vi "Elevator Control.vi"(11 "Shooter Elevation PID Gains":T1={"proportional gain (Kc)"=2.5, "integral time (Ti, min)"=0.0, "derivative time (Td, min)"=0.0003} {"derivative time (Td, min)" format="%.5f"; "integral time (Ti, min)" format="%.3f"; "proportional gain (Kc)" format="%.3f"}) -> (2 "Shooter Pot Setpoint":dbl=3.84, 3 "Elevator Output":dbl=-0.06325507999999869)   [LabVIEW 2012]
uses:
  Globals/Shooter Elevation Positons.vi
  Globals/Useful Values.vi
  <vilib>/Rock Robotics/WPI/Joystick/WPI_JoystickGetSetRefNum.vi
  Robot Global Data.vi
  Globals/Log Data.vi
  <vilib>/addons/control/pid/pid.llb/PID (DBL).vi
  <vilib>/addons/control/pid/NI_PID_pid.lvlib
panel:
  out "Shooter Pot Voltage":dbl
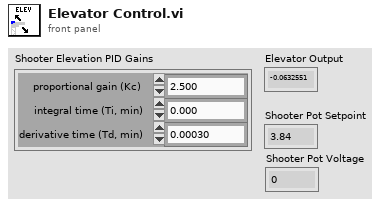
[diagram p1: front panel]
types:
  T1 = cluster{"proportional gain (Kc)":dbl, "integral time (Ti, min)":dbl, "derivative time (Td, min)":dbl}
  T2 = typedef "WPI_AnalogChannelDevRef.ctl" = cluster{"DevStatus":errorcluster, "Analog Module":T3, "Analog Channel":T4}
  T3 = typedef "FPGA_TypedefAnalogModule.ctl" = enum16{"Analog Module 1", "Analog Module 2"}
  T4 = typedef "FPGA_AIChannel.ctl" = enum8{"AI 1", "AI 2", "AI 3", "AI 4", "AI 5", "AI 6", "AI 7", "AI 8", "Invalid"}
  T5 = typedef "WPI_MotorControlDeviceRef.ctl" = cluster{"DeviceStatus":errorcluster, "Type":enum16{"PWM", "CAN"}, "PWM":cluster{"Digital Module":T6, "PWM Channel":T7, "DeadBand":T8}, "CAN":cluster{"Device Number":u8, "Control Mode":T9, "Semaphore":T10, "Max Vout":dbl}, "Invert":bool, "TransformRef":T11, "InvTransformRef":T11}
  T6 = typedef "FPGA_TypedefDigitalModule.ctl" = enum16{"Digital Module 1", "Digital Module 2"}
  T7 = typedef "FPGA_DIOPWMChannel.ctl" = enum8{"PWM 1", "PWM 2", "PWM 3", "PWM 4", "PWM 5", "PWM 6", "PWM 7", "PWM 8", "PWM 9", "PWM 10", "Invalid"}
  T8 = typedef "WPI_PWMDeadband.ctl" = cluster{"Name":string, "maxPositivePwm":i32, "minPositivePwm":i32, "centerPwm":i32, "maxNegativePwm":i32, "minNegativePwm":i32, "angularRange":u16}
  T9 = typedef "WPI_CANJaguar_ControlMode.ctl" = enum8{"Percent VBus", "Current", "Speed", "Position", "Voltage"}
  T10 = typedef "Semaphore RefNum" = refnum<k1>
  T11 = typedef "WPI_PWMTransform_ConPane.ctl" = refnum<vi>
  T12 = typedef "WPI_JoystickDevRef.ctl" = cluster{"Device":T13}
  T13 = typedef "WPI_JoystickDeviceEnum.ctl" = enum16{"USB 1", "USB 2", "USB 3", "USB 4", "Kinect 1", "Kinect 2"}
  T14 = typedef "WPI_JoystickButtonState.ctl" = cluster{"Button 1":bool, "Button 2":bool, "Button 3":bool, "Button 4":bool, "Button 5":bool, "Button 6":bool, "Button 7":bool, "Button 8":bool, "Button 9":bool, "Button 10":bool, "Button 11":bool, "Button 12":bool}
  T15 = typedef "WPI_DriverStationRobotMode2.ctl" = enum16{"Autonomous Disabled", "Autonomous Enabled", "Teleop Disabled", "Teleop Enabled", "Timeout", "Finish", "Test Disabled", "Test Enabled"}
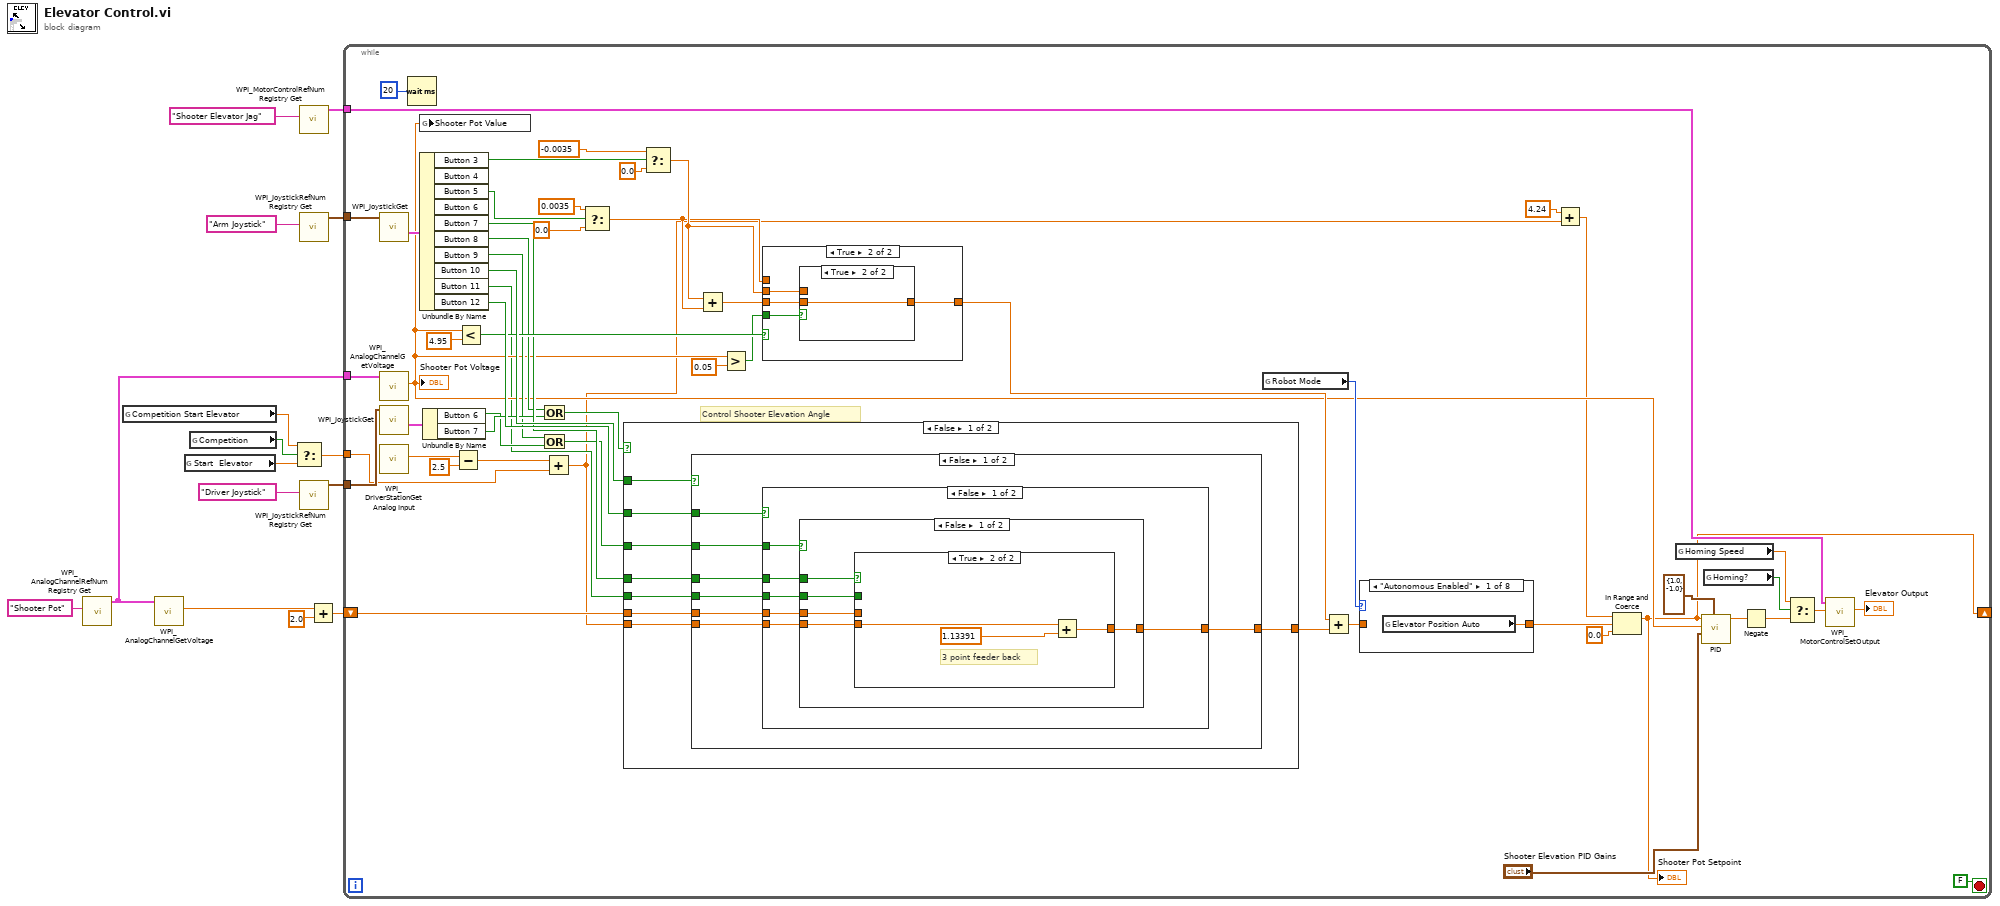
[diagram p0: block diagram]
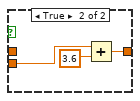
[diagram p12: hidden frame]
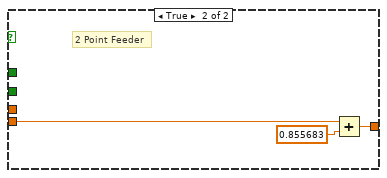
[diagram p13: hidden frame]
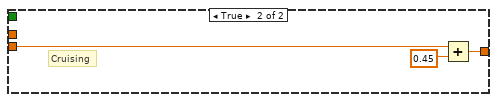
[diagram p14: hidden frame]
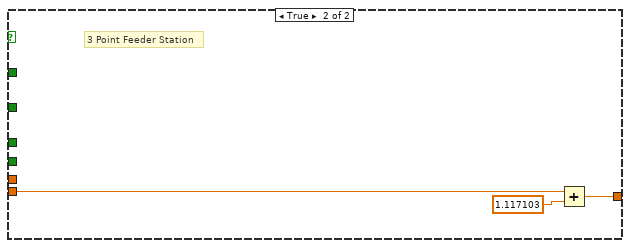
[diagram p15: hidden frame]
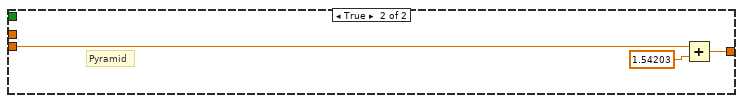
[diagram p16: hidden frame]
diagram:
  n1 = call <vilib>:"WPI_AnalogChannelRefNum Registry Get.vi"("refnum name"="Shooter Pot") -> ("AIDeviceRef"=w4:T2)  [unwired: 9 in, 1 out]
  n2 = global read "Shooter Elevation Positons.vi" "Competition Start Elevator"() -> (w14:dbl)
  n3 = call <vilib>:"WPI_AnalogChannelGetVoltage.vi"("AIDeviceRef"=w4) -> ("Voltage"=w2:dbl)  [unwired: 8 in, 2 out]
  n4 = global read "Shooter Elevation Positons.vi" "Start  Elevator"() -> (w12:dbl)
  n5 = global read "Useful Values.vi" "Competition"() -> (w13:bool)
  n6 = Select(t=w14, s=w13, f=w12) -> (s? t:f=w15:dbl)
  n7 = call <vilib>:"WPI_MotorControlRefNum Registry Get.vi"("refnum name"="Shooter Elevator Jag") -> ("MotorControlDevRef"=w7:T5)  [unwired: 9 in, 1 out]
  n8 = call <vilib>:"WPI_JoystickRefNum Registry Get.vi"("refnum name"="Arm Joystick") -> ("JoystickDevRef"=w9:T12)  [unwired: 9 in, 1 out]
  n9 = call <vilib>:"WPI_JoystickRefNum Registry Get.vi"("refnum name"="Driver Joystick") -> ("JoystickDevRef"=w5:T12)  [unwired: 9 in, 1 out]
  n10 = Add(x=w2, y=2.0) -> (x+y=w3:dbl)
  n11 = while {
    tunnel: w4 -> [w65]
    tunnel: w9 -> [w68]
    tunnel: w7 -> [w43]
    shift-right: [w22] -> _
    shift-left: w3 -> [w60]
    tunnel: w15 -> [w17]
    tunnel: w5 -> [w39]
    stop <- FALSE stop-if-true
    # "Control Shooter Elevation Angle"
    n12 = call <vilib>:"WPI_JoystickGet.vi"("JoystickDevRef"=w68) -> ("Buttons"=w64:T14)  [unwired: 1 in, 5 out]
    n13 = call <vilib>:"WPI_AnalogChannelGetVoltage.vi"("AIDeviceRef"=w65) -> ("Voltage"=w27:dbl)  [unwired: 8 in, 2 out]
    "Shooter Pot Voltage" <- w27
    n14 = call <vilib>:"WPI_JoystickGet.vi"("JoystickDevRef"=w39) -> ("Buttons"=w38:T14)  [unwired: 1 in, 5 out]
    n15 = call <vilib>:"WPI_DriverStationGet Analog Input.vi"() -> ("Analog 2 (V)"=w19:dbl)  [unwired: 8 in, 3 out]
    n16 = Wait (ms)(milliseconds to wait=u32 20) -> ()  [unwired: 1 out]
    n17 = global write "Log Data.vi" "Shooter Pot Value"(w27) -> ()
    n18 = Unbundle By Name(w64) -> ("Button 3"=w52:bool, "Button 5"=w57:bool, "Button 7"=w42:bool, "Button 8"=w37:bool, "Button 9"=w33:bool, "Button 10"=w62:bool, "Button 11"=w21:bool, "Button 12"=w63:bool)  [unwired: 2 out]
    n19 = Unbundle By Name(w38) -> ("Button 6"=w34:bool, "Button 7"=w36:bool)
    n20 = Subtract(x=w19, y=2.5) -> (x-y=w18:dbl)
    n21 = Less?(x=w27, y=4.95) -> (x < y?=w49:bool)
    n22 = Or(x=w37, y=w36) -> (x .or. y?=w35:bool)
    n23 = Or(x=w33, y=w34) -> (x .or. y?=w32:bool)
    n24 = Add(x=w18, y=w17) -> (x+y=w16:dbl)
    n25 = Select(t=0.0035, s=w57, f=0.0) -> (s? t:f=w46:dbl)
    n26 = case shown="False" w35 {
      tunnel: [w93 w134] -> w58
      tunnel: w62 -> [w92 _]
      tunnel: w63 -> [w91 _]
      tunnel: w60 -> [w90 _]
      tunnel: w42 -> [w89 _]
      tunnel: w32 -> [w88 _]
      tunnel: w16 -> [w87 w132]
      tunnel: w21 -> [w86 _]
      frame False {
        n27 = case shown="False" w92 {
          tunnel: [w100 w130] -> w93
          tunnel: w91 -> [w99 _]
          tunnel: w90 -> [w98 _]
          tunnel: w89 -> [w97 _]
          tunnel: w88 -> [w96 _]
          tunnel: w87 -> [w95 w129]
          tunnel: w86 -> [w94 _]
          frame False {
            n28 = case shown="False" w99 {
              tunnel: [w104 w128] -> w100
              tunnel: w98 -> [w105 _]
              tunnel: w97 -> [w102 _]
              tunnel: w96 -> [w106 _]
              tunnel: w95 -> [w103 w126]
              tunnel: w94 -> [w101 _]
              frame False {
                n29 = case shown="False" w106 {
                  tunnel: w105 -> [w108 _]
                  tunnel: [w110 w124] -> w104
                  tunnel: w103 -> [w109 w123]
                  tunnel: w102 -> [w111 _]
                  tunnel: w101 -> [w107 _]
                  frame False {
                    n30 = case shown="True" w111 {
                      tunnel: [w113 w122] -> w110
                      tunnel: w109 -> [w112 w120]
                      tunnel: w108 -> [w114 _]
                      tunnel: w107 -> [w115 _]
                      frame False {
                        n31 = case shown="False" w115 {
                          tunnel: w114 -> [w116 _]
                          tunnel: [w116 w117] -> w113
                          tunnel: w112 -> [_ w119]
                          frame False {
                          }
                          frame True {
                            n32 = Add(x=w119, y=3.6) -> (x+y=w117:dbl)
                          }
                        }
                      }
                      frame True {
                        # "3 point feeder back"
                        n33 = Add(x=w120, y=1.13391) -> (x+y=w122:dbl)
                      }
                    }
                  }
                  frame True {
                    # "2 Point Feeder"
                    n34 = Add(x=w123, y=0.855683) -> (x+y=w124:dbl)
                  }
                }
              }
              frame True {
                # "Cruising"
                n35 = Add(x=w126, y=0.45) -> (x+y=w128:dbl)
              }
            }
          }
          frame True {
            # "3 Point Feeder Station"
            n36 = Add(x=w129, y=1.117103) -> (x+y=w130:dbl)
          }
        }
      }
      frame True {
        # "Pyramid"
        n37 = Add(x=w132, y=1.54203) -> (x+y=w134:dbl)
      }
    }
    n38 = Select(t=-0.0035, s=w52, f=0.0) -> (s? t:f=w47:dbl)
    n39 = Add(x=w47, y=w46) -> (x+y=w44:dbl)
    n40 = Greater?(x=w27, y=0.05) -> (0:w48:bool)
    n41 = case shown="True" w49 {
      tunnel: w48 -> [_ w80]
      tunnel: w46 -> [w79 _]
      tunnel: [w79 w83] -> w45
      tunnel: w47 -> [_ w81]
      tunnel: w44 -> [_ w82]
      frame False {
      }
      frame True {
        n42 = case shown="True" w80 {
          tunnel: [w84 w85] -> w83
          tunnel: w82 -> [_ w85]
          tunnel: w81 -> [w84 _]
          frame False {
          }
          frame True {
          }
        }
      }
    }
    n43 = global read "Robot Global Data.vi" "Robot Mode"() -> (w41:T15)
    n44 = Add(x=w45, y=w58) -> (x+y=w40:dbl)
    n45 = case shown="\"Autonomous Enabled\"" w41 {
      tunnel: w40 -> [_ w72 w73 w74 w75 w76 w77 w78]
      tunnel: [w71 w72 w73 w74 w75 w76 w77 w78] -> w23
      frame "Autonomous Enabled" {
        n46 = global read "Useful Values.vi" "Elevator Position Auto"() -> (w71:dbl)
      }
      frame "Teleop Enabled" {
      }
      frame "Timeout" {
      }
      frame "Finish" {
      }
      frame "Test Disabled" {
      }
      frame "Test Enabled" {
      }
      frame "Teleop Disabled" {
      }
      frame "Autonomous Disabled" {
      }
    }
    n47 = Add(x=4.24 ("lower limit"), y=w16) -> (x+y=w24:dbl)
    n48 = In Range and Coerce(upper limit=w24, x=w23, lower limit=0.0) -> (coerced(x)=w22:dbl)  [unwired: 1 out]
    "Shooter Pot Setpoint" <- w22
    n49 = global read "Useful Values.vi" "Homing Speed"() -> (w29:dbl)
    n50 = call-poly <vilib>:"PID.vi"("output range"=cluster{"output high":dbl, "output low":dbl} {"output high"=1.0, "output low"=-1.0}, "PID gains"="Shooter Elevation PID Gains", "process variable"=w27, "setpoint"=w22) -> ("output"=w59:dbl)  [unwired: 6 in, 1 out]
    n51 = global read "Useful Values.vi" "Homing?"() -> (w31:bool)
    n52 = Negate(x=w59) -> (-x=w30:dbl)
    n53 = Select(t=w29, s=w31, f=w30) -> (s? t:f=w28:dbl)
    n54 = call <vilib>:"WPI_MotorControlSetOutput.vi"("Output"=w28, "MotorControlDevRef"=w43) -> ("Motor Output"=→"Elevator Output":dbl)  [unwired: 7 in, 2 out]
  }
